vi "resource entries to table.vi"(7 "Sort Type":T3 items=["RIO device", "resource", "input type", "datatype", "reserver"], 8 "error in (no error)":errorcluster, 10 "resource entries":T1[](array[typedef]) {"FPGA CD Ref" format="%.0x"; "reserver" format="%.0x"}) -> (0 "error out":errorcluster, 1 "sorted resource table out":string[][](array[string]), 2 "sorted resource entries out":T1[](array[typedef]) {"FPGA CD Ref" format="%.0x"; "reserver" format="%.0x"})   [LabVIEW 2016, in "FPGA Resource Manager.lvlib"]
uses:
  FPGA Resource Manager.lvlib
  resource info.ctl
  <vilib>/NI Veristand/Custom Device API/Custom Device Item Ref.ctl
  viz_type.ctl
  <vilib>/NI VeriStand/Custom Device API/Custom Device API.lvlib
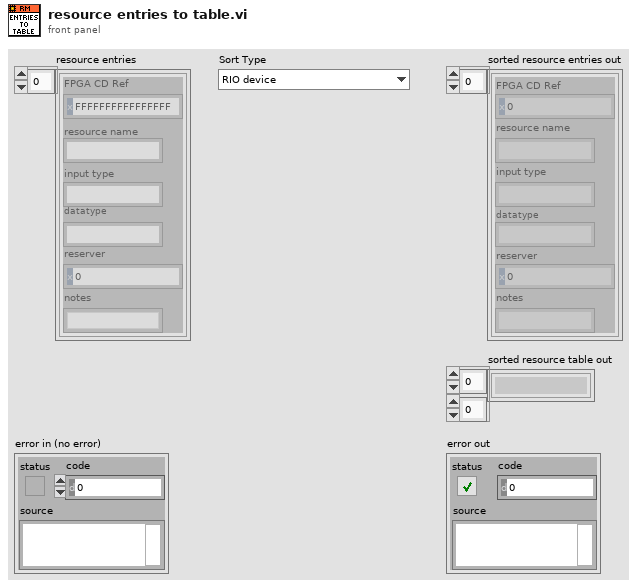
[diagram p1: front panel]
types:
  T1 = typedef "FPGA Resource Manager.lvlib/resource info.ctl" = cluster{"FPGA CD Ref":T2, "resource name":string, "input type":string, "datatype":string, "reserver":T2, "notes":string}
  T2 = typedef "Custom Device API.lvlib/Custom Device Item Ref.ctl" = u64
  T3 = typedef "FPGA Resource Manager.lvlib/viz_type.ctl" = u16
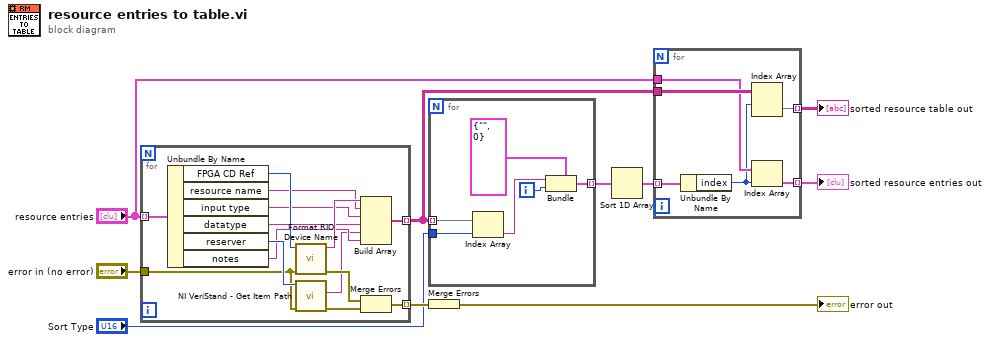
[diagram p0: block diagram]
diagram:
  n1 = for {
    tunnel: "resource entries" -> [w24] mode=indexing
    tunnel: [w23] -> w3 mode=indexing
    tunnel: "error in (no error)" -> [w18]
    tunnel: [w17] -> w9 mode=indexing
    n2 = Unbundle By Name(w24) -> ("FPGA CD Ref"=w22:T2, "resource name"=w15:string, "input type"=w14:string, "datatype"=w11:string, "reserver"=w21:T2, "notes"=w13:string)
    n3 = call "Format RIO Device Name.vi"("error in (no error)"=w18, "FPGA CD Ref"=w22) -> ("error out"=w20:errorcluster, "String"=w16:string)  [unwired: 8 in]
    n4 = call <vilib>:"NI VeriStand - Get Item Path.vi"("error in (no error)"=w18, "Item Ref in"=w21) -> ("error out"=w19:errorcluster, "Path"=w12:string)  [unwired: 6 in, 2 out]
    n5 = Build Array(w16, w15, w14, w11, w12, w13) -> (w23:string[])
    n6 = Merge Errors(w20, w19) -> (w17:errorcluster)
  }
  n7 = for {
    tunnel: w3 -> [w27] mode=indexing
    tunnel: "Sort Type" -> [w26]
    tunnel: [w29] -> w6 mode=indexing
    i -> [w30]
    n8 = Index Array(array=w27, index=w26) -> (element=w25:string)
    n9 = Bundle(cluster=cluster{"key":string, "index":i32} {"key"="", "index"=0}, "key"=w25, "index"=w30) -> (w29:cluster{"key":string, "index":i32})
  }
  n10 = Merge Errors(w9) -> (→"error out":errorcluster)
  n11 = Sort 1D Array(array=w6) -> (sorted array=w5:cluster{"key":string, "index":i32}[])
  n12 = for {
    tunnel: w5 -> [w36] mode=indexing
    tunnel: w3 -> [w35]
    tunnel: [w34] -> w4 mode=indexing
    tunnel: "resource entries" -> [w33]
    tunnel: [w32] -> w1 mode=indexing
    n13 = Unbundle By Name(w36) -> ("index"=w31:i32)
    n14 = Index Array(array=w35, index (row)=w31) -> (element=w34:string[])  [unwired: 1 in]
    n15 = Index Array(array=w33, index=w31) -> (element=w32:T1)
  }
  "sorted resource table out" <- w4
  "sorted resource entries out" <- w1
